vi "error_handling.vi"(8 "error in (no error)":errorcluster, 10 "error handle":i32, 11 "object in":refnum<class "SQLiteConnection.lvclass">) -> (0 "error out":errorcluster, 3 "object out":refnum<class "SQLiteConnection.lvclass">)   [LabVIEW 2019, in "SQLiteConnection.lvclass"]
uses:
  SQLiteConnection.lvclass
  <vilib>/Utility/error.llb/DialogType.ctl
  SQLiteConnection.lvclass/SQLiteConnection.ctl
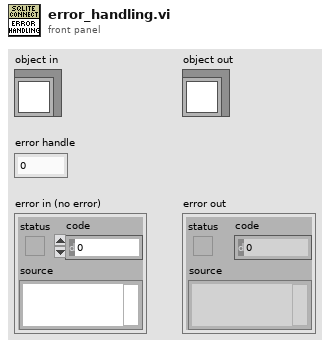
[diagram p1: front panel]
types:
  T1 = typedef "DialogType.ctl" = u16
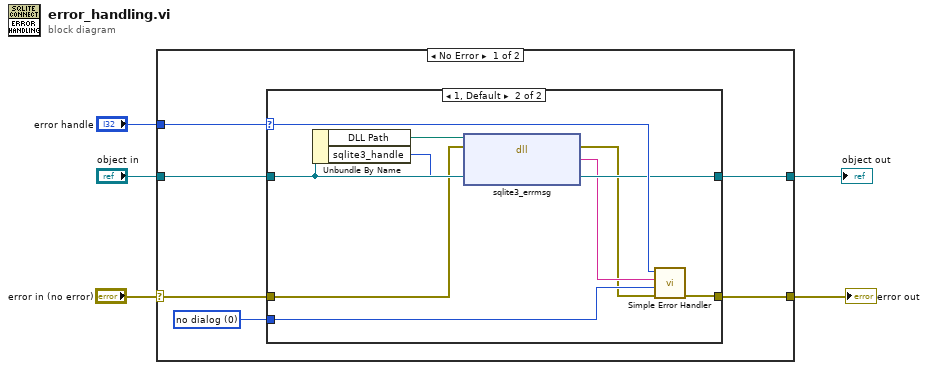
[diagram p0: block diagram]
diagram:
  n1 = case shown="No Error" "error in (no error)" {
    selector: "error in (no error)" -> [w10 w24]
    tunnel: "error handle" -> [w11 _]
    tunnel: [w9 w24] -> w3
    tunnel: "object in" -> [w7 w23]
    tunnel: [w6 w23] -> w1
    frame No Error {
      w8 = T1 0 items=["no dialog", "OK message", "continue or stop message", "OK message + warnings", "continue/stop + warnings"] ("type of dialog (OK msg:1)")
      n2 = case shown="1, Default" w11 {
        selector: w11 -> [_ w21]
        tunnel: w10 -> [w13 w17]
        tunnel: [w13 w22] -> w9
        tunnel: w8 -> [_ w20]
        tunnel: w7 -> [w12 w19]
        tunnel: [w12 w19] -> w6
        frame 0, 100, 101 {
          # "SQLITE_OK\nSQLITE_DONE\nSQLITE_ROW"
        }
        frame 1, Default {
          (unwired) "" ("message")
          (unwired) "G" ("message")
          n3 = Unbundle By Name(w19) -> ("DLL Path"=w18:path, "sqlite3_handle"=w16:u64)
          n4 = dll-call lib="D:/Users/mcarl/Documents/LabVIEW Projects/OW-PIKO/OW-PIKO Software/sqlite3.dll" fn="sqlite3_errmsg"(path in=w18, error in=w17, "sqlit3_handle"=w16) -> (error out=w14:errorcluster, "return type"=w15:string)  [unwired: 2 in, 1 out]
          n5 = call <vilib>:"Simple Error Handler.vi"("error code (no error:0)"=w21, "error source (\" \")"=w15, "type of dialog (OK msg:1)"=w20, "error in (no error)"=w14) -> ("error out"=w22:errorcluster)  [unwired: 1 in, 4 out]
        }
      }
    }
    frame Error {
    }
  }
  "error out" <- w3
  "object out" <- w1
